vi "Get Default HTTP Client Implementation.vi"() -> (3 "HTTP Client Abstract out":refnum<class "Abstract HTTP Client.lvclass">)   [LabVIEW 2020, in "HTTP Client Abstract.lvlib" / "Abstract HTTP Client.lvclass"]
uses:
  Abstract HTTP Client.lvclass
  LabVIEW HTTP Client/LabVIEW HTTP Client.lvclass
  C:/Projects/http-client-plugin-base/lv_src/Classes/LabVIEW HTTP Client/LabVIEW HTTP Client.lvclass
  C:/Projects/http-client-plugin-base/lv_src/Classes/Abstract HTTP Client/Abstract HTTP Client.lvclass
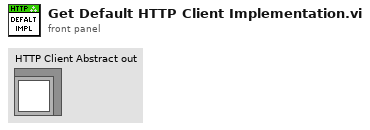
[diagram p1: front panel]
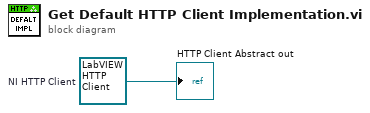
[diagram p0: block diagram]
diagram:
  w1 = refnum<class "LabVIEW HTTP Client.lvclass"> refnum  # NI HTTP Client
  "HTTP Client Abstract out" <- w1
